vi "receiveData.vi"(8 "error in (no error)":errorcluster, 11 "Model in":refnum<class "Model.lvclass">) -> (0 "error out":errorcluster, 3 "Model out":refnum<class "Model.lvclass">)   [LabVIEW 2013, in "Model.lvclass"]
uses:
  Model.lvclass
  <userlib>/Common/ILC/ILC/ILC.lvclass
  <userlib>/Common/Devices/ForceSensorCalculator/ForceSensorCalculator/ForceSensorCalculator.lvclass
  Typedefs/ForceDemand.ctl
  Typedefs/FAMTTypedefs.lvlib
  Typedefs/InputData.ctl
  UserEvents/UserEvents.lvclass
  ApplicationElements/Log/TestDataLog/TestDataLog.lvclass
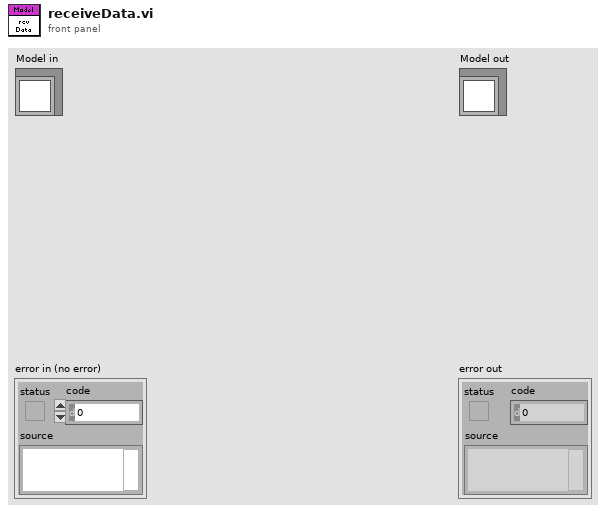
[diagram p1: front panel]
types:
  T1 = typedef "FAMTTypedefs.lvlib/InputData.ctl" = cluster{"Force Measured":T2}
  T2 = typedef "FAMTTypedefs.lvlib/ForceDemand.ctl" = dbl[unit]
  T3 = typedef "FAMTTypedefs.lvlib/PubDataEvents.ctl" = cluster{"State":refnum<user-event>, "ErrorCode":refnum<user-event>, "OutputData":refnum<user-event>, "InputData":refnum<user-event>, "ControllerData":refnum<user-event>, "TestStatus":refnum<user-event>, "LogPath":refnum<user-event>}
  T4 = typedef "ILCCommon.lvlib/ILCTypedefs.lvlib/ADCsInEngineeringUnits.ctl" = cluster{"Ch1":dbl[unit], "Ch2":dbl[unit], "Ch3":dbl[unit], "Ch4":dbl[unit]}
  T5 = typedef "ILCCommon.lvlib/ILCTypedefs.lvlib/InputData.ctl" = cluster{"Input Channels":T6, "Limit Switches":T7, "Tachometer":u16, "SSI Encoder":i32, "ADCs":T8}
  T6 = typedef "ILCCommon.lvlib/ILCConfiguration.lvlib/InputChannels.ctl" = enum16{"Channel 0", "3 Channels", "5 Channels"}
  T7 = typedef "ILCCommon.lvlib/ILCTypedefs.lvlib/LimitSwitches.ctl" = cluster{"1":bool, "2":bool}
  T8 = typedef "ILCCommon.lvlib/ILCTypedefs.lvlib/ADCs.ctl" = cluster{"Ch0":i32, "Ch1":i32, "Ch2":i32, "Ch3":i32, "Ch4":i32}
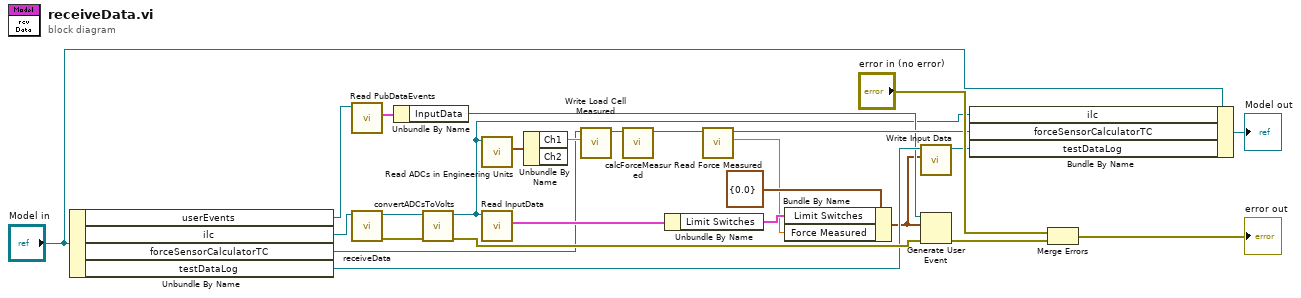
[diagram p0: block diagram]
diagram:
  n1 = Unbundle By Name("Model in") -> ("userEvents"=w9:refnum<class "UserEvents.lvclass">, "ilc"=w4:refnum<class "ILC.lvclass">, "forceSensorCalculatorTC"=w1:refnum<class "ForceSensorCalculatorTC.lvclass">, "testDataLog"=w12:refnum<class "TestDataLog.lvclass">)
  n2 = call "Read PubDataEvents.vi"("UserEvents in"=w9) -> ("PubDataEvents"=w5:T3)  [unwired: 9 in, 1 out]
  n3 = call <userlib>:"receiveData.vi"("ILC in"=w4) -> ("error out"=w20:errorcluster, "ILC out"=w21:refnum<class "ILC.lvclass">)  [unwired: 9 in]
  n4 = Unbundle By Name(w5) -> ("InputData"=w10:refnum<user-event>)
  n5 = call <userlib>:"convertADCsToVolts.vi"("error in (no error)"=w20, "ILC in"=w21) -> ("error out"=w19:errorcluster, "ILC out"=w8:refnum<class "ILC.lvclass">)  [unwired: 8 in]
  n6 = call <userlib>:"Read ADCs in Engineering Units.vi"("ILC in"=w8) -> ("ADCs in Engineering Units"=w18:T4)  [unwired: 9 in, 1 out]
  n7 = call <userlib>:"Read InputData.vi"("ILC in"=w8) -> ("InputData"=w14:T5)  [unwired: 9 in, 1 out]
  n8 = Unbundle By Name(w18) -> ("Ch1"=w3:dbl[unit])  [unwired: 1 out]
  n9 = call <userlib>:"Write Load Cell Measured.vi"("Load Cell Measured"=w3, "ForceSensor in"=w1) -> ("ForceSensor out"=w2:refnum<class "ForceSensorCalculatorTC.lvclass">)  [unwired: 9 in]
  n10 = call <userlib>:"calcForceMeasured.vi"("ForceSensor in"=w2) -> ("ForceSensor out"=w17:refnum<class "ForceSensorCalculatorTC.lvclass">)  [unwired: 9 in, 1 out]
  n11 = Unbundle By Name(w14) -> ("Limit Switches"=w13:T7)
  n12 = call <userlib>:"Read Force Measured.vi"("ForceSensor in"=w17) -> ("Force Demand"=w6:dbl[unit], "ForceSensor out"=w16:refnum<class "ForceSensorCalculatorTC.lvclass">)  [unwired: 9 in]
  n13 = Bundle By Name(cluster=T1 {"Force Measured"=0.0} ("event data"), "Limit Switches"=w13, "Force Measured"=w6) -> (w7:T1)
  n14 = call "Write Input Data.vi"("Input Data"=w7, "Logger in"=w12) -> ("Logger out"=w11:refnum<class "TestDataLog.lvclass">)  [unwired: 9 in]
  n15 = Generate User Event(user event=w10, event data cluster=w7, error in=w19) -> (error out=w23:errorcluster)  [unwired: 1 in, 1 out]
  n16 = Bundle By Name(cluster="Model in", "ilc"=w8, "forceSensorCalculatorTC"=w16, "testDataLog"=w11) -> (→"Model out":refnum<class "Model.lvclass">)
  n17 = Merge Errors("error in (no error)", w23) -> (→"error out":errorcluster)
